vi "TiposdeDatos.vi"() -> ()   [LabVIEW 2020]
panel:
  out "Tank":u8(slide) scale=0.0..10.0
  in  "Dial":u8(knob) scale=0.0..10.0
  out "Thermometer":dbl(slide) scale=0.0..100.0
  in  "Knob":dbl(knob) scale=0.0..10.0
  # "Tipos de Datos"
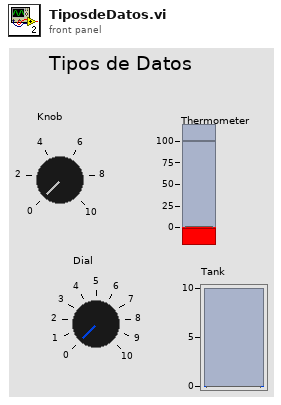
[diagram p1: front panel]
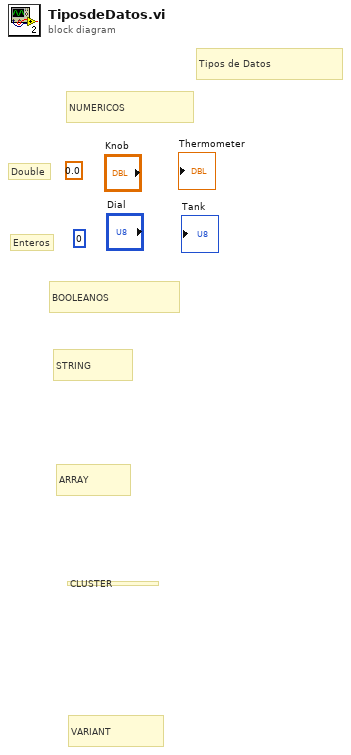
[diagram p0: block diagram]
diagram:
  (unwired) 0
  (unwired) 0.0
  # "Enteros"
  # "Double"
  # "VARIANT"
  # "CLUSTER"
  # "ARRAY"
  # "STRING"
  # "BOOLEANOS"
  # "NUMERICOS"
  # "Tipos de Datos"
